vi "myRIO_BRig_Host_v0,32.vi"() -> ()   [LabVIEW 2014]
panel:
  out "error_LoadPrevSettings":errorcluster caption="error out"
  in  "LoadPrevSettings":bool
  out "graph_ai1":dbl(graph)
  out "graph_ai0":dbl(graph)
  in  "dataIn_maxTrialsDisplayed":i32 caption="Number of Trials Displayed\n( 0 = all trials )"
  out "error_TCP":errorcluster
  in  "stop":bool
  in  "colorIn_timeout":u32(colorbox)=7468543 caption="Choice Timeout"
  in  "colorIn_wrong/cue":u32(colorbox)=16728618 caption="Wrong Choice or\nLicked During Cue"
  in  "colorIn_reward":u32(colorbox)=5898088 caption="Reward"
  in  "colorIn_unknown":u32(colorbox)=16449331 caption="Unknown Trial Status"
  out "dataOut_plot":cluster{i32[], i32[]}[](graph)
  out "iTrial":i32
  out "iBlock":i32
  # "Exp Stats"
  # "Current Block Stats"
  # "Trials 2 Reward\n\nBad Trials\nPost Reward"
  # "Left Spout    Right Spout"
  # "Run Time\n\n   minutes    seconds"
  # "Average Block Stats"
  # "Trials 2 Reward\n\nBad Trials\nPost Reward"
  # "Left Spout    Right Spout"
  # "If you get ERROR 5 related to opening a file, press CONTINUE"
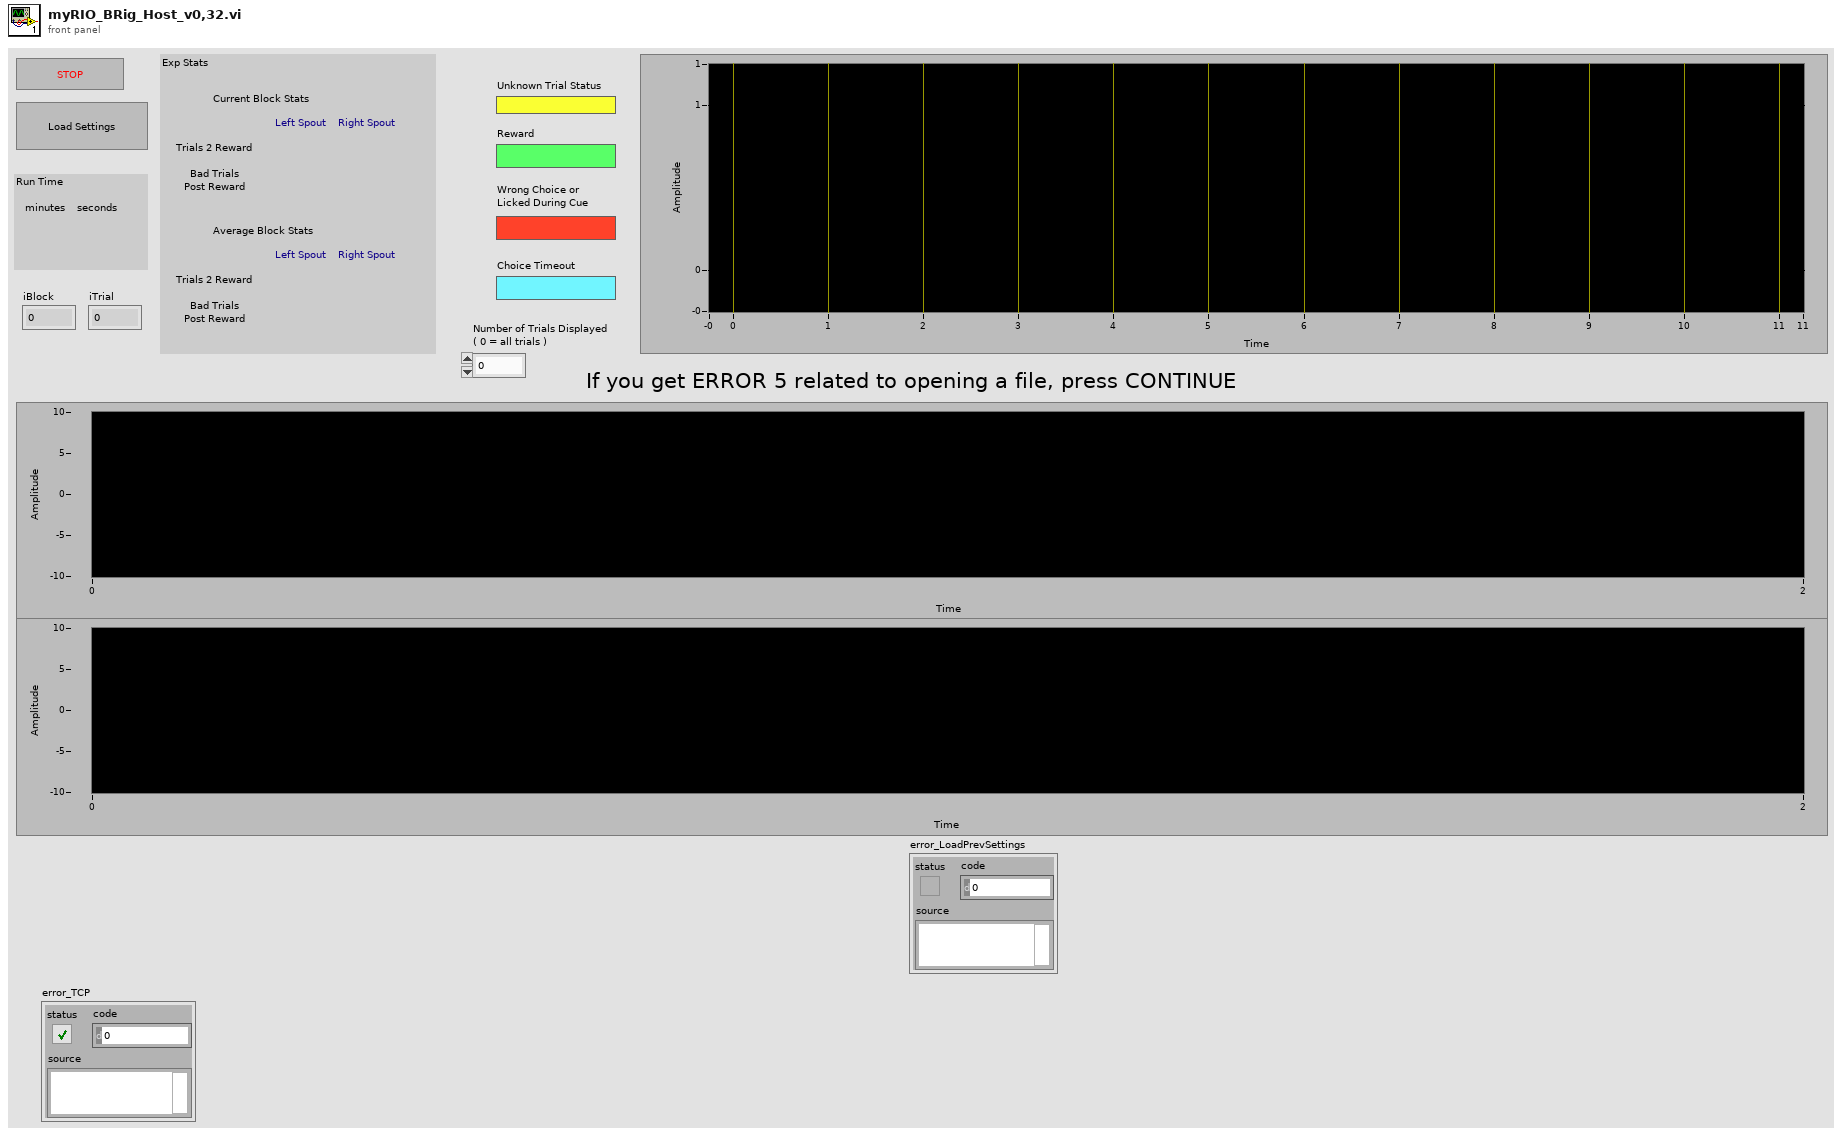
[diagram p1: front panel]
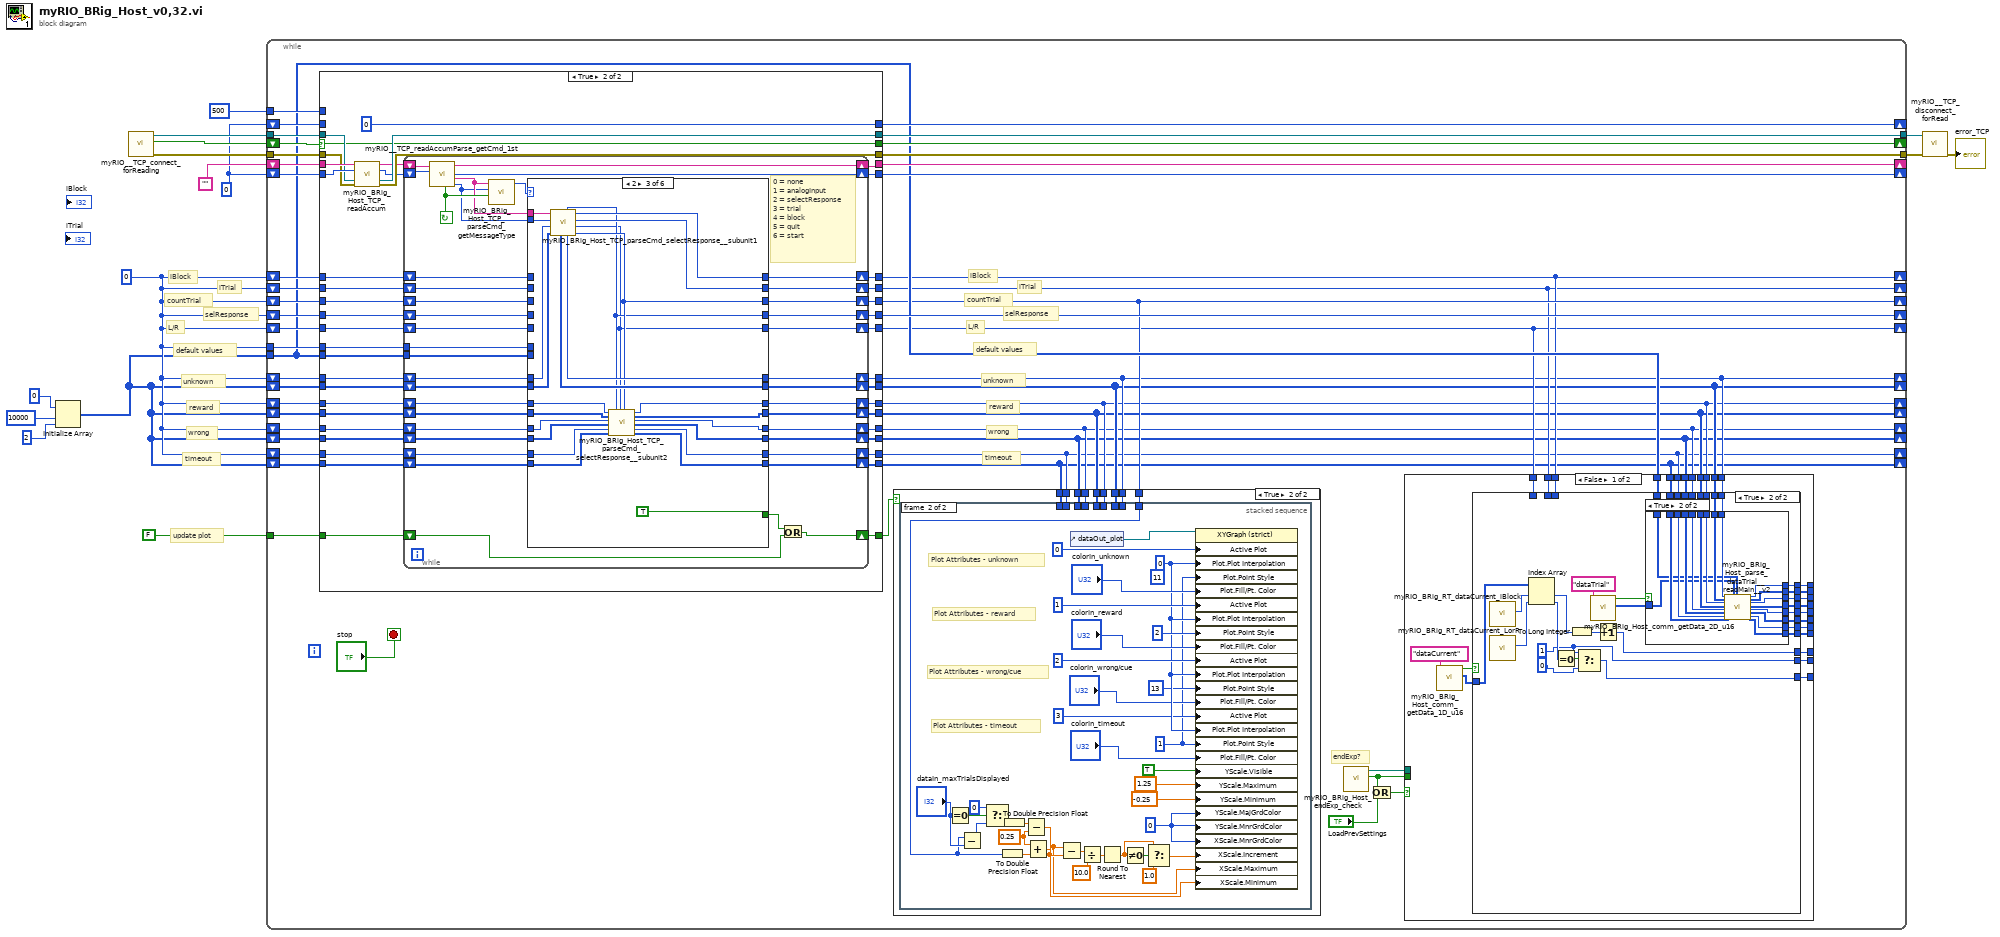
[diagram p0: block diagram]
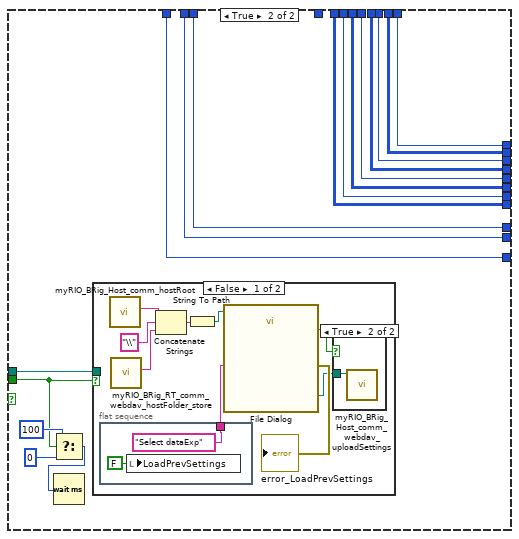
[diagram p4: hidden frame]
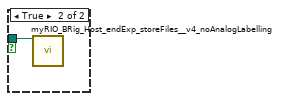
[diagram p6: hidden frame]
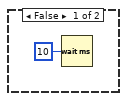
[diagram p7: hidden frame]
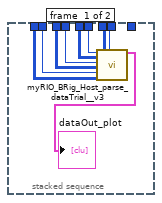
[diagram p8: hidden frame]
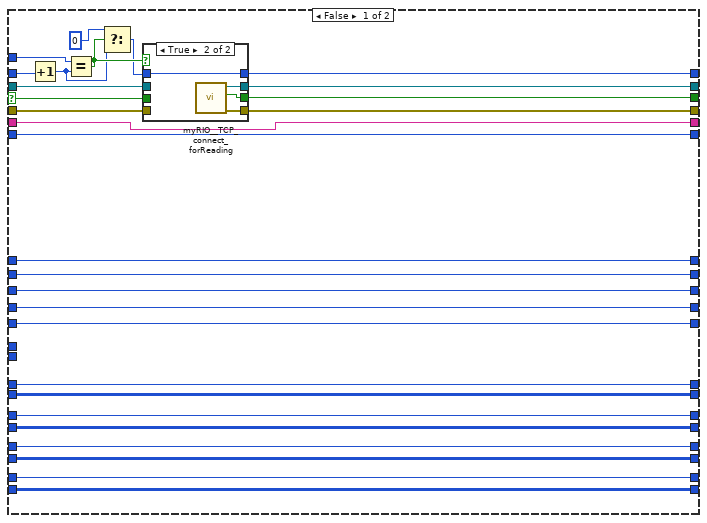
[diagram p9: hidden frame]
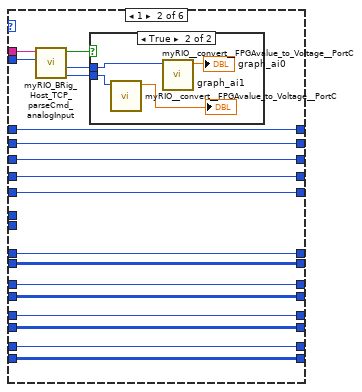
[diagram p12: hidden frame]
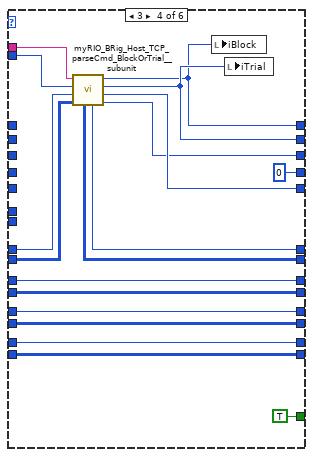
[diagram p14: hidden frame]
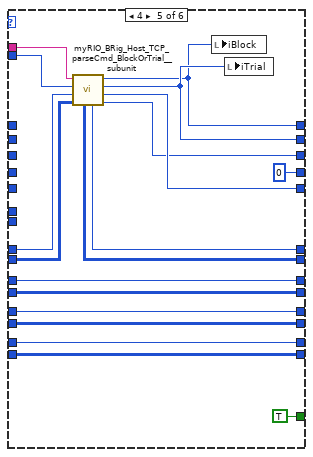
[diagram p15: hidden frame]
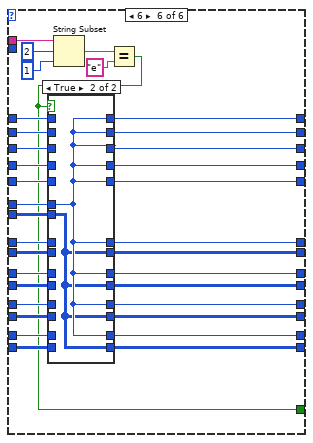
[diagram p16: hidden frame]
diagram:
  w2 = 0
  w11 = 0
  # "default values"
  # "update plot"
  # "timeout"
  # "wrong"
  # "reward"
  # "unknown"
  # "L/R"
  # "selResponse"
  # "countTrial"
  # "iBlock"
  # "iTrial"
  n1 = Initialize Array(0 ("element"), 10000 ("dimension size"), 2 ("dimension size")) -> (w1:i32[][])
  n2 = call "myRIO__TCP_connect_forReading.vi"() -> ("output_error"=w13:errorcluster, "output_connected"=w14:bool, "output_hTCP"=w15:refnum<k5>)  [unwired: 9 in]
  n3 = while {
    tunnel: w15 -> [w62]
    tunnel: w13 -> [w60]
    shift-right: [w53] -> _
    shift-left: w11 -> [w58]
    shift-right: [w54] -> _
    shift-left: "" -> [w59]
    shift-right: [w55] -> _
    shift-left: w14 -> [w61]
    shift-right: [w56] -> _
    shift-left: w11 -> [w63]
    tunnel: 500 ("y") -> [w57]
    shift-right: [w26] -> _
    shift-left: w2 -> [w52]
    shift-right: [w25] -> _
    shift-left: w2 -> [w51]
    shift-right: [w27] -> _
    shift-left: w2 -> [w50]
    shift-right: [w38] -> _
    shift-left: w2 -> [w49]
    shift-right: [w24] -> _
    shift-left: w2 -> [w48]
    shift-right: [w23] -> _
    shift-left: w2 -> [w47]
    shift-right: [w22] -> _
    shift-left: w1 -> [w46]
    shift-right: [w21] -> _
    shift-left: w2 -> [w45]
    shift-right: [w20] -> _
    shift-left: w1 -> [w44]
    shift-right: [w19] -> _
    shift-left: w2 -> [w43]
    shift-right: [w18] -> _
    shift-left: w1 -> [w42]
    shift-right: [w17] -> _
    shift-left: w2 -> [w41]
    shift-right: [w16] -> _
    shift-left: w1 -> [w40]
    tunnel: [w36] -> w5
    tunnel: [w35] -> w4
    tunnel: FALSE -> [w39]
    tunnel: w2 -> [w33]
    tunnel: w1 -> [w28]
    stop <- "stop" stop-if-true
    # "default values"
    # "timeout"
    # "wrong"
    # "reward"
    # "unknown"
    # "L/R"
    # "selResponse"
    # "countTrial"
    # "iBlock"
    # "iTrial"
    # "endExp?"
    n4 = case shown="True" w61 {
      selector: w61 -> [w263 w312]
      tunnel: w59 -> [w257 w318]
      tunnel: w58 -> [w258 w317]
      tunnel: [w257 w308] -> w54
      tunnel: [w258 w307] -> w53
      tunnel: w62 -> [w264 w316]
      tunnel: [w267 w315] -> w36
      tunnel: w60 -> [w262 w314]
      tunnel: [w266 w313] -> w35
      tunnel: [w265 w312] -> w55
      tunnel: w63 -> [w268 _]
      tunnel: [w256 0] -> w56
      tunnel: w57 -> [w255 _]
      tunnel: w52 -> [w254 w306]
      tunnel: w51 -> [w253 w305]
      tunnel: w50 -> [w252 w304]
      tunnel: w49 -> [w251 w303]
      tunnel: w48 -> [w250 w302]
      tunnel: w47 -> [w249 w301]
      tunnel: w46 -> [w248 w300]
      tunnel: w45 -> [w247 w299]
      tunnel: w44 -> [w246 w298]
      tunnel: w43 -> [w245 w297]
      tunnel: w42 -> [w244 w296]
      tunnel: w41 -> [w243 w295]
      tunnel: w40 -> [w242 w294]
      tunnel: w39 -> [_ w293]
      tunnel: [_ w292] -> w37
      tunnel: [w254 w291] -> w26
      tunnel: [w253 w290] -> w25
      tunnel: [w252 w289] -> w27
      tunnel: [w251 w288] -> w38
      tunnel: [w250 w287] -> w24
      tunnel: [w249 w286] -> w23
      tunnel: [w248 w285] -> w22
      tunnel: [w247 w284] -> w21
      tunnel: [w246 w283] -> w20
      tunnel: [w245 w282] -> w19
      tunnel: [w244 w281] -> w18
      tunnel: [w243 w280] -> w17
      tunnel: [w242 w279] -> w16
      tunnel: w33 -> [_ w278]
      tunnel: w28 -> [_ w277]
      frame False {
        n5 = Increment(x=w268) -> (x+1=w241:i32)
        n6 = Equal?(x=w255, y=w241) -> (x = y?=w261:bool)
        n7 = Select(t=0, s=w261, f=w241) -> (s? t:f=w259:i32)
        n8 = case shown="True" w261 {
          tunnel: w259 -> [w269 w273]
          tunnel: [w272 w276] -> w267
          tunnel: [w270 w275] -> w266
          tunnel: [w271 w274] -> w265
          tunnel: w264 -> [w272 _]
          tunnel: w263 -> [w271 _]
          tunnel: w262 -> [w270 _]
          tunnel: [w269 w273] -> w256
          frame False {
          }
          frame True {
            n9 = call "myRIO__TCP_connect_forReading.vi"() -> ("output_error"=w275:errorcluster, "output_connected"=w274:bool, "output_hTCP"=w276:refnum<k5>)  [unwired: 9 in]
          }
        }
      }
      frame True {
        n10 = call "myRIO_BRig_Host_TCP_readAccum.vi"("input_strAccum"=w318, "input_count"=w317, "input_handle_TCP"=w316, "input_error"=w314) -> ("output_strAccum"=w310:string, "output_count"=w309:i32, "output_handle_TCP"=w315:refnum<k5>, "output_error"=w313:errorcluster)  [unwired: 8 in]
        n11 = while {
          shift-right: [w355] -> w308
          shift-left: w310 -> [w357]
          shift-right: [w354] -> w307
          shift-left: w309 -> [w356]
          shift-right: [w346] -> w291
          shift-left: w306 -> [w349]
          shift-right: [w345] -> w290
          shift-left: w305 -> [w348]
          shift-right: [w344] -> w289
          shift-left: w304 -> [w347]
          shift-right: [w342] -> w288
          shift-left: w303 -> [w343]
          shift-right: [w340] -> w287
          shift-left: w302 -> [w341]
          shift-right: [w338] -> w286
          shift-left: w301 -> [w339]
          shift-right: [w336] -> w285
          shift-left: w300 -> [w337]
          shift-right: [w329] -> w284
          shift-left: w299 -> [w335]
          shift-right: [w328] -> w283
          shift-left: w298 -> [w334]
          shift-right: [w327] -> w282
          shift-left: w297 -> [w333]
          shift-right: [w326] -> w281
          shift-left: w296 -> [w332]
          shift-right: [w324] -> w279
          shift-left: w294 -> [w330]
          shift-right: [w325] -> w280
          shift-left: w295 -> [w331]
          shift-right: [w322] -> w292
          shift-left: w293 -> [w319]
          tunnel: w278 -> [w321]
          tunnel: w277 -> [w320]
          stop <- w353 continue-if-true
          # "0 = none\n1 = analogInput\n2 = selectResponse\n3 = trial\n4 = block\n5 = quit\n6 = start"
          n12 = call "myRIO__TCP_readAccumParse_getCmd_1st.vi"("input_count"=w356, "input_strAccum"=w357) -> ("output_countCmd"=w351:i32, "output_strCmd"=w352:string, "output_count"=w354:i32, "output_strAccum"=w355:string, "output_haveCmd"=w353:bool)  [unwired: 5 in]
          n13 = call "myRIO_BRig_Host_TCP_parseCmd_getMessageType.vi"("input_haveCmd"=w353, "input_countCmd"=w351, "input_strCmd"=w352) -> ("output_messageType"=w350:u8)  [unwired: 8 in]
          n14 = case shown="2" w350 {
            tunnel: w352 -> [_ w375 w416 w433 w451 w486]
            tunnel: w351 -> [_ w374 w415 w432 w450 _]
            tunnel: w349 -> [w370 w388 _ _ _ w481]
            tunnel: w348 -> [w369 w387 _ _ _ w479]
            tunnel: w347 -> [w368 w386 _ _ _ w478]
            tunnel: [w370 w388 w410 w418 w436 w480] -> w346
            tunnel: [w369 w387 w409 w419 w437 w475] -> w345
            tunnel: [w368 w386 w408 w426 w444 w474] -> w344
            tunnel: w343 -> [w367 w385 _ _ _ w477]
            tunnel: [w367 w385 w407 0 ("output_iTrial_num") 0 ("output_iTrial_num") w473] -> w342
            tunnel: w341 -> [w366 w384 _ _ _ w476]
            tunnel: [w366 w384 w406 w427 w445 w472] -> w340
            tunnel: w339 -> [w365 w383 w414 w431 w449 w471]
            tunnel: [w365 w383 w412 w429 w447 w463] -> w338
            tunnel: w337 -> [w364 w382 w413 w430 w448 w470]
            tunnel: [w364 w382 w411 w428 w446 w462] -> w336
            tunnel: w335 -> [w363 w381 w405 w425 w443 w469]
            tunnel: w334 -> [w362 w380 w404 w424 w442 w468]
            tunnel: w333 -> [w361 w379 w403 w423 w441 w467]
            tunnel: w332 -> [w360 w378 w402 w422 w440 w466]
            tunnel: w331 -> [w359 w377 w401 w421 w439 w465]
            tunnel: w330 -> [w358 w376 w400 w420 w438 w464]
            tunnel: [w363 w381 w399 w425 w443 w461] -> w329
            tunnel: [w362 w380 w398 w424 w442 w460] -> w328
            tunnel: [w361 w379 w397 w423 w441 w459] -> w327
            tunnel: [w360 w378 w396 w422 w440 w458] -> w326
            tunnel: [w359 w377 w395 w421 w439 w457] -> w325
            tunnel: [w358 w376 w394 w420 w438 w456] -> w324
            tunnel: [_ _ TRUE TRUE TRUE w453] -> w323
            tunnel: w321 -> [_ _ _ _ _ w455]
            tunnel: w320 -> [_ _ _ _ _ w454]
            frame 0, Default {
            }
            frame 1 {
              n15 = call "myRIO_BRig_Host_TCP_parseCmd_analogInput.vi"("input_countCmd"=w374, "input_strCmd"=w375) -> ("output_ai1"=w371:i32, "output_ai0"=w372:i32, "output_haveAnalogInput"=w373:bool)  [unwired: 7 in]
              n16 = case shown="True" w373 {
                tunnel: w372 -> [_ w392]
                tunnel: w371 -> [_ w390]
                frame False {
                }
                frame True {
                  n17 = call "myRIO__convert__FPGAvalue_to_Voltage__PortC.vi"("input_FPGAvalue_PortC"=w390) -> ("output_voltage"=→"graph_ai1":dbl)  [unwired: 10 in]
                  n18 = call "myRIO__convert__FPGAvalue_to_Voltage__PortC.vi"("input_FPGAvalue_PortC"=w392) -> ("output_voltage"=→"graph_ai0":dbl)  [unwired: 10 in]
                }
              }
            }
            frame 2 {
              n19 = call "myRIO_BRig_Host_TCP_parseCmd_selectResponse__subunit1.vi"("input_arrayUnknown"=w413, "input_idxUnknown"=w414, "input_countCmd"=w415, "input_strCmd"=w416) -> ("output_countTrial"=w408:i32, "output_L/R"=w406:i32, "output_iTrial"=w409:i32, "output_iBlock"=w410:i32, "output_idxUnknown"=w412:i32, "output_response"=w407:i32, "output_arrayUnknown"=w411:i32[][])  [unwired: 1 in]
              n20 = call "myRIO_BRig_Host_TCP_parseCmd_selectResponse__subunit2.vi"("input_idxReward"=w405, "input_arrayReward"=w404, "input_idxWrong"=w403, "input_arrayWrong"=w402, "input_idxTimeout"=w401, "input_arrayTimeout"=w400, "input_response"=w407, "input_L/R"=w406, "input_countTrial"=w408) -> ("output_idxReward"=w399:i32, "output_arrayReward"=w398:i32[][], "output_idxWrong"=w397:i32, "output_arrayWrong"=w396:i32[][], "output_idxTimeout"=w395:i32, "output_arrayTimeout"=w394:i32[][])  [unwired: 5 in]
            }
            frame 3 {
              n21 = call "myRIO_BRig_Host_TCP_parseCmd_BlockOrTrial__subunit.vi"("input_arrayUnknown"=w430, "input_idxUnknown"=w431, "input_countCmd"=w432, "input_strCmd"=w433) -> ("output_countTrial"=w426:i32, "output_L/R"=w427:i32, "output_iTrial"=w419:i32, "output_iBlock"=w418:i32, "output_idxUnknown"=w429:i32, "output_arrayUnknown"=w428:i32[][])  [unwired: 2 in]
              n22 = local write "iBlock"(w418) -> ()
              n23 = local write "iTrial"(w419) -> ()
            }
            frame 4 {
              n24 = call "myRIO_BRig_Host_TCP_parseCmd_BlockOrTrial__subunit.vi"("input_arrayUnknown"=w448, "input_idxUnknown"=w449, "input_countCmd"=w450, "input_strCmd"=w451) -> ("output_countTrial"=w444:i32, "output_L/R"=w445:i32, "output_iTrial"=w437:i32, "output_iBlock"=w436:i32, "output_idxUnknown"=w447:i32, "output_arrayUnknown"=w446:i32[][])  [unwired: 2 in]
              n25 = local write "iBlock"(w436) -> ()
              n26 = local write "iTrial"(w437) -> ()
            }
            frame 6 {
              n27 = String Subset(string=w486, offset (0)=2, length (rest)=1 ("length (rest)")) -> (substring=w483:string)
              n28 = Equal?(x=w483, y="e") -> (x = y?=w453:bool)
              n29 = case shown="True" w453 {
                tunnel: w481 -> [w499 _]
                tunnel: [w499 w501] -> w480
                tunnel: w479 -> [w498 _]
                tunnel: w478 -> [w497 _]
                tunnel: w477 -> [w496 _]
                tunnel: w476 -> [w495 _]
                tunnel: [w498 w501] -> w475
                tunnel: [w497 w501] -> w474
                tunnel: [w496 w501] -> w473
                tunnel: [w495 w501] -> w472
                tunnel: w471 -> [w494 _]
                tunnel: w470 -> [w493 _]
                tunnel: w469 -> [w492 _]
                tunnel: w468 -> [w491 _]
                tunnel: w467 -> [w490 _]
                tunnel: w466 -> [w489 _]
                tunnel: w465 -> [w488 _]
                tunnel: w464 -> [w487 _]
                tunnel: [w494 w501] -> w463
                tunnel: [w493 w500] -> w462
                tunnel: [w492 w501] -> w461
                tunnel: [w491 w500] -> w460
                tunnel: [w490 w501] -> w459
                tunnel: [w489 w500] -> w458
                tunnel: [w488 w501] -> w457
                tunnel: [w487 w500] -> w456
                tunnel: w455 -> [_ w501]
                tunnel: w454 -> [_ w500]
                frame False {
                }
                frame True {
                }
              }
            }
          }
          n30 = Or(x=w323, y=w319) -> (x .or. y?=w322:bool)
        }
      }
    }
    n31 = case shown="True" w37 {
      tunnel: w16 -> [_ w196]
      tunnel: w17 -> [_ w195]
      tunnel: w18 -> [_ w194]
      tunnel: w19 -> [_ w193]
      tunnel: w20 -> [_ w192]
      tunnel: w21 -> [_ w191]
      tunnel: w22 -> [_ w190]
      tunnel: w23 -> [_ w189]
      tunnel: w27 -> [_ w188]
      frame False {
        n32 = Wait (ms)(milliseconds to wait=u32 10) -> ()  [unwired: 1 out]
      }
      frame True {
        n33 = stacked-sequence {
          tunnel: w196 -> [w205 _]
          tunnel: w195 -> [w204 _]
          tunnel: w194 -> [w203 _]
          tunnel: w193 -> [w202 _]
          tunnel: w192 -> [w201 _]
          tunnel: w191 -> [w200 _]
          tunnel: w190 -> [w199 _]
          tunnel: w189 -> [w198 _]
          tunnel: w188 -> [_ w214]
          frame #0 {
            n34 = call "myRIO_BRig_Host_parse_dataTrial__v3.vi"("input_idxReward"=w200, "input_arrayReward"=w201, "input_idxWrong"=w202, "input_arrayWrong"=w203, "input_idxTimeout"=w204, "input_arrayTimeout"=w205, "input_arrayUnknown"=w199, "input_idxUnknown"=w198) -> ("output_plotData"=→"dataOut_plot":cluster{i32[], i32[]}[])  [unwired: 11 in]
          }
          frame #1 {
            w210 = u32 0 ("Y Scale.Grid Colors:Major Color")
            w218 = 0.25 ("y")
            w207 = u8 1 ("Plot.Point Style")
            (unwired) u8 11 ("Plot.Point Style")
            w234 = u8 0 ("Plot.Plot Interpolation")
            # "Plot Attributes - timeout"
            # "Plot Attributes - wrong/cue"
            # "Plot Attributes - reward"
            # "Plot Attributes - unknown"
            n35 = Equal To 0?(x="dataIn_maxTrialsDisplayed") -> (x = 0?=w215:bool)
            n36 = Subtract(x=w214, y="dataIn_maxTrialsDisplayed") -> (x-y=w216:i32)
            n37 = Select(t=0, s=w215, f=w216) -> (s? t:f=w221:i32)
            n38 = To Double Precision Float(number=w214) -> (double precision float=w219:dbl)
            n39 = To Double Precision Float(number=w221) -> (double precision float=w220:dbl)
            n40 = Subtract(x=w220, y=w218) -> (x-y=w208:dbl)
            n41 = Add(x=w218, y=w219) -> (x+y=w206:dbl)
            n42 = Subtract(x=w206, y=w208) -> (x-y=w222:dbl)
            n43 = control-ref of="dataOut_plot"() -> (w229:refnum<vi>)
            n44 = Divide(x=w222, y=10.0) -> (x/y=w224:dbl)
            n45 = Round To Nearest(number=w224) -> (nearest integer value=w226:dbl)
            n46 = Not Equal To 0?(x=w226) -> (x != 0?=w225:bool)
            n47 = Select(t=w226, s=w225, f=1.0) -> (s? t:f=w209:dbl)
            n48 = property on="Property Node" class="XYGraph (strict)"(reference=w229, "Active Plot"=u32 0, "Plot.Plot Interpolation"=w234, "Plot.Point Style"=w207, "Plot.Fill/Pt. Color"="colorIn_unknown", "Active Plot"=u32 1, "Plot.Plot Interpolation"=w234, "Plot.Point Style"=u8 2, "Plot.Fill/Pt. Color"="colorIn_reward", "Active Plot"=u32 2, "Plot.Plot Interpolation"=w234, "Plot.Point Style"=u8 13, "Plot.Fill/Pt. Color"="colorIn_wrong/cue", "Active Plot"=u32 3, "Plot.Plot Interpolation"=w234, "Plot.Point Style"=w207, "Plot.Fill/Pt. Color"="colorIn_timeout", "YScale.Visible"=TRUE ("Y Scale.Visible"), "YScale.Maximum"=1.25 ("Y Scale.Range:Maximum"), "YScale.Minimum"=-0.25 ("Y Scale.Range:Minimum"), "YScale.MajGrdColor"=w210, "YScale.MnrGrdColor"=w210, "XScale.MnrGrdColor"=w210, "XScale.Increment"=w209, "XScale.Maximum"=w206, "XScale.Minimum"=w208) -> ()  [unwired: 1 in, 2 out]
          }
        }
      }
    }
    n49 = call "myRIO_BRig_Host_endExp_check.vi"() -> ("output_IendExp"=w30:bool, "output_filePath_expExp"=w29:path)  [unwired: 10 in]
    n50 = Or(x=w30, y="LoadPrevSettings") -> (x .or. y?=w31:bool)
    n51 = case shown="False" w31 {
      tunnel: w30 -> [_ w170]
      tunnel: w29 -> [_ w169]
      tunnel: [w86 w168] -> _
      tunnel: [w85 w167] -> _
      tunnel: [w84 w166] -> _
      tunnel: [w83 w165] -> _
      tunnel: [w82 w164] -> _
      tunnel: [w81 w163] -> _
      tunnel: [w80 w162] -> _
      tunnel: [w79 w161] -> _
      tunnel: w23 -> [w78 w168]
      tunnel: w22 -> [w77 w167]
      tunnel: w21 -> [w76 w166]
      tunnel: w20 -> [w75 w165]
      tunnel: w19 -> [w74 w164]
      tunnel: w18 -> [w73 w163]
      tunnel: w17 -> [w72 w162]
      tunnel: w16 -> [w71 w161]
      tunnel: w28 -> [w70 _]
      tunnel: [w69 w158] -> _
      tunnel: [w68 w159] -> _
      tunnel: [w67 w160] -> _
      tunnel: w26 -> [w66 w160]
      tunnel: w25 -> [w65 w159]
      tunnel: w24 -> [w64 w158]
      frame False {
        n52 = call "myRIO_BRig_Host_comm_getData_1D_u16.vi"("input_fileName"="dataCurrent") -> ("output_data_1D"=w87:u16[], "output_I_data"=w88:bool)  [unwired: 9 in]
        n53 = case shown="True" w88 {
          tunnel: w87 -> [_ w131]
          tunnel: [w100 w126] -> w86
          tunnel: [w99 w125] -> w85
          tunnel: [w98 w124] -> w84
          tunnel: [w97 w123] -> w83
          tunnel: [w96 w122] -> w82
          tunnel: [w95 w121] -> w81
          tunnel: [w94 w120] -> w80
          tunnel: [w93 w119] -> w79
          tunnel: w78 -> [w100 w118]
          tunnel: w77 -> [w99 w117]
          tunnel: w76 -> [w98 w116]
          tunnel: w75 -> [w97 w115]
          tunnel: w74 -> [w96 w114]
          tunnel: w73 -> [w95 w113]
          tunnel: w72 -> [w94 w112]
          tunnel: w71 -> [w93 w111]
          tunnel: w70 -> [_ w110]
          tunnel: [w90 w106] -> w69
          tunnel: [w91 w105] -> w68
          tunnel: [w92 w101] -> w67
          tunnel: w66 -> [w92 _]
          tunnel: w65 -> [w91 _]
          tunnel: w64 -> [w90 _]
          frame False {
          }
          frame True {
            w105 = 1
            n54 = call "myRIO_BRig_RT_dataCurrent_iBlock.vi"() -> ("output_iBlock"=w104:i32)  [unwired: 11 in]
            n55 = call "myRIO_BRig_RT_dataCurrent_LorR.vi"() -> ("output_LorR"=w127:i32)  [unwired: 11 in]
            n56 = Index Array(array=w131, index #1=w104, index #2=w127) -> (element #1=w103:u16, element #2=w109:u16)
            n57 = Equal To 0?(x=w109) -> (x = 0?=w108:bool)
            n58 = To Long Integer(number=w103) -> (32bit integer=w102:i32)
            n59 = Select(t=w105, s=w108, f=0) -> (s? t:f=w106:i32)
            n60 = call "myRIO_BRig_Host_comm_getData_2D_u16.vi"("input_fileName"="dataTrial") -> ("output_data_2D"=w128:u16[][], "output_I_data"=w129:bool)  [unwired: 9 in]
            n61 = Increment(x=w102) -> (x+1=w101:i32)
            n62 = case shown="True" w129 {
              tunnel: w128 -> [_ w149]
              tunnel: [w137 w145] -> w124
              tunnel: [w136 w144] -> w123
              tunnel: [w138 w146] -> w125
              tunnel: [w139 w147] -> w126
              tunnel: [w135 w143] -> w122
              tunnel: [w134 w142] -> w121
              tunnel: [w133 w141] -> w120
              tunnel: [w132 w140] -> w119
              tunnel: w110 -> [_ w148]
              tunnel: w118 -> [w139 w157]
              tunnel: w117 -> [w138 w156]
              tunnel: w116 -> [w137 w155]
              tunnel: w115 -> [w136 w154]
              tunnel: w114 -> [w135 w153]
              tunnel: w113 -> [w134 w152]
              tunnel: w112 -> [w133 w151]
              tunnel: w111 -> [w132 w150]
              frame False {
              }
              frame True {
                n63 = call "myRIO_BRig_Host_parse_dataTrial__readMain__v2.vi"("input_idxUnknown"=w157, "input_arrayUnknown"=w156, "input_idxReward"=w155, "input_arrayReward"=w154, "input_idxWrong"=w153, "input_arrayWrong"=w152, "input_idxTimeout"=w151, "input_arrayTimeout"=w150, "arrayIn_dataTrial"=w149, "arrayIn_empty"=w148) -> ("output_idxUnknown"=w147:i32, "output_arrayUnknown"=w146:i32[][], "output_idxReward"=w145:i32, "output_arrayReward"=w144:i32[][], "output_idxWrong"=w143:i32, "output_arrayWrong"=w142:i32[][], "output_idxTimeout"=w141:i32, "output_arrayTimeout"=w140:i32[][])  [unwired: 10 in]
              }
            }
          }
        }
      }
      frame True {
        n64 = Select(t=u32 100 ("milliseconds to wait"), s=w170, f=u32 0 ("milliseconds to wait")) -> (s? t:f=w172:u32)
        n65 = Wait (ms)(milliseconds to wait=w172) -> ()  [unwired: 1 out]
        n66 = case shown="False" w170 {
          tunnel: w169 -> [_ w186]
          frame False {
            n67 = flat-sequence {
              tunnel: ["Select dataExp" ("prompt")] -> w177
              frame #0 {
                n68 = local write "LoadPrevSettings"(FALSE ("LoadPrevSettings")) -> ()
              }
            }
            n69 = call "myRIO_BRig_Host_comm_hostRoot.vi"() -> ("output_hostRoot"=w179:string)  [unwired: 11 in]
            n70 = call "myRIO_BRig_RT_comm_webdav_hostFolder_store.vi"() -> ("output_HostFolder"=w181:string)  [unwired: 11 in]
            n71 = Concatenate Strings(w179, "\\" ("string"), w181) -> (w182:string)
            n72 = String To Path(string=w182) -> (path=w178:path)
            n73 = call "File Dialog"("start path"=w178, "prompt"=w177) -> ("selected path"=w174:path, "exists"=w175:bool, "error out"=→"error_LoadPrevSettings":errorcluster)  [unwired: 10 in, 1 out]
            n74 = case shown="True" w175 {
              tunnel: w174 -> [_ w183]
              frame False {
              }
              frame True {
                n75 = call "myRIO_BRig_Host_comm_webdav_uploadSettings.vi"("input_filePath"=w183) -> ()  [unwired: 11 in]
              }
            }
          }
          frame True {
            n76 = call "myRIO_BRig_Host_endExp_storeFiles__v4_noAnalogLabelling.vi"("input_filePath"=w186) -> ()  [unwired: 15 in]
          }
        }
      }
    }
  }
  n77 = call "myRIO__TCP_disconnect_forRead.vi"("input_error"=w4, "input_hTCP"=w5) -> ("output_error"=→"error_TCP":errorcluster)  [unwired: 9 in]
